vi "Demo - QuickDrop.vi"() -> ()   [LabVIEW 2020]
uses:
  <vilib>/ErrorRing/Error Ring.xnode
  <vilib>/Analysis/NI_AALBase.lvlib
panel:
  in  "error in (no error) 2":errorcluster
  out "error out 7":errorcluster
  in  "Numeric 4":dbl
  in  "String 4":string
  out "Numeric 3":dbl
  out "String 3":string
  out "error out 6":errorcluster
  out "error out 5":errorcluster
  out "error out 4":errorcluster
  out "error out 3":errorcluster
  out "error out 2":errorcluster
  out "String 2":string
  out "Numeric 2":dbl
  in  "String":string
  in  "Numeric":dbl
  out "error out":errorcluster
  in  "error in (no error)":errorcluster
  # "LabVIEW QuickDrop"
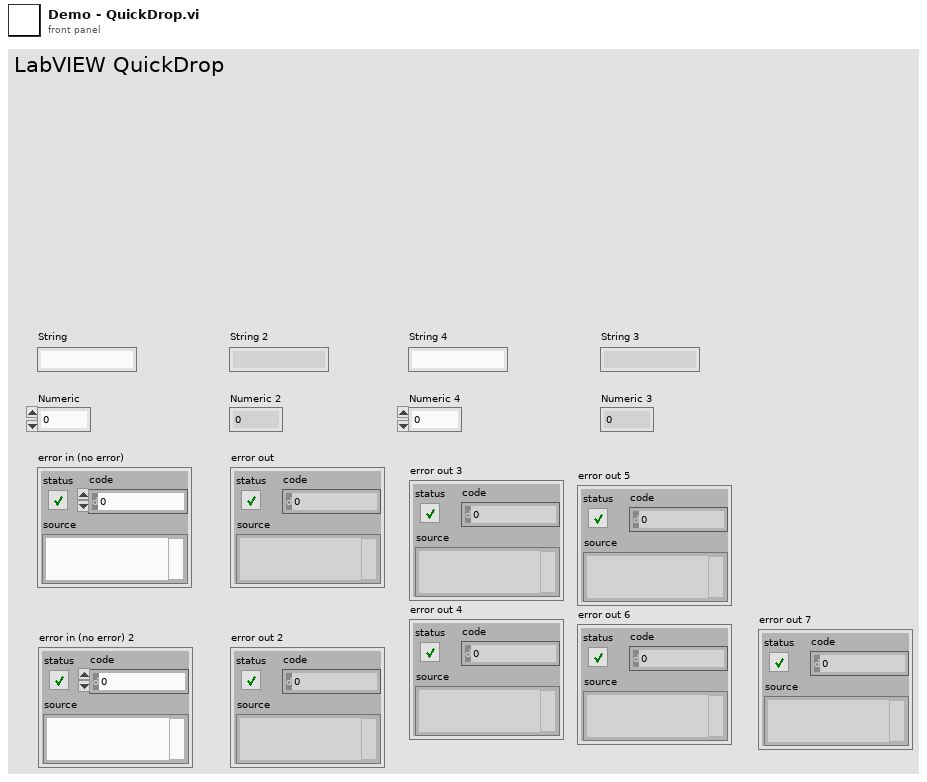
[diagram p1: front panel]
types:
  T1 = enum16{"QD - Wire ctrl & ind", "QD - Wire constants", "QD - FP Reorder as pane connector", "QD - Wire multiple lines", "QD - Wire multiple and cleanup", "QD - Remove item", "QD - Remove unconnected items from bbn", "QD - Reposition labels and icons", "QD - Replace items", "QD - Insert one wire or all wires", "QD - VI Server class rename", "QD - Property method selection", "QD - FP BD to Origin", "QD - Icon Creation", "QD- Combination - Replacing td controls FP", "QD- Combination - Replacing td controls BD"}
  T2 = cluster{"Num 1":i32, "Num 2":i32, "Num 3":i32, "Num 4":i32, "Num 5":i32}
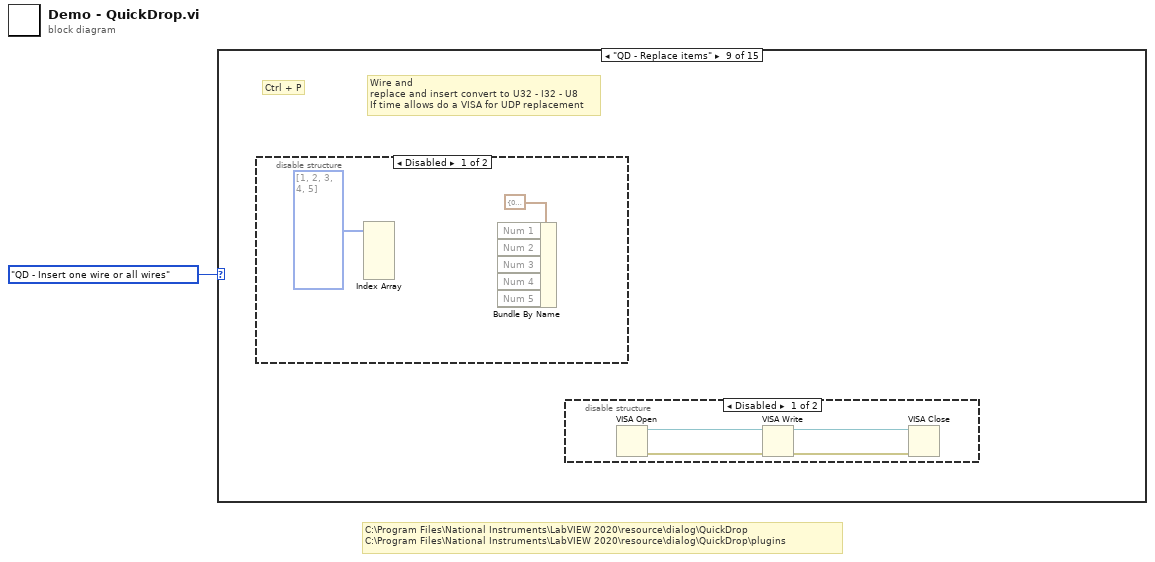
[diagram p0: block diagram]
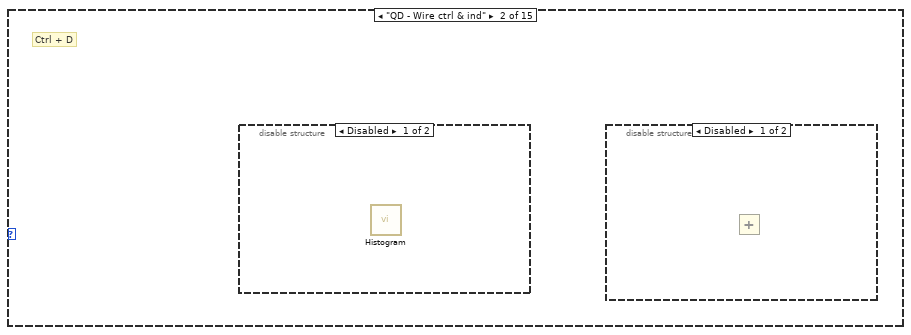
[diagram p3: hidden frame]
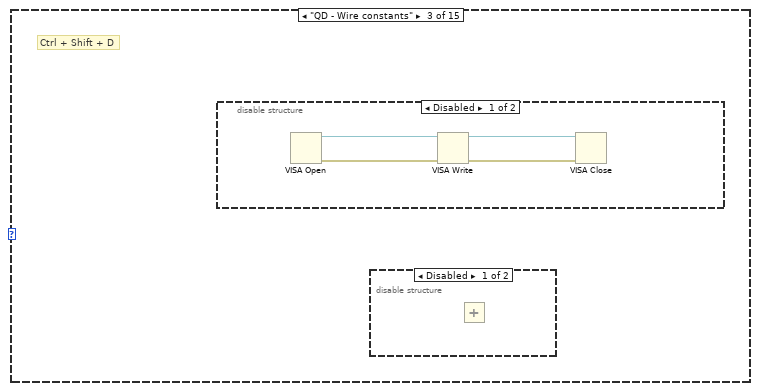
[diagram p6: hidden frame]
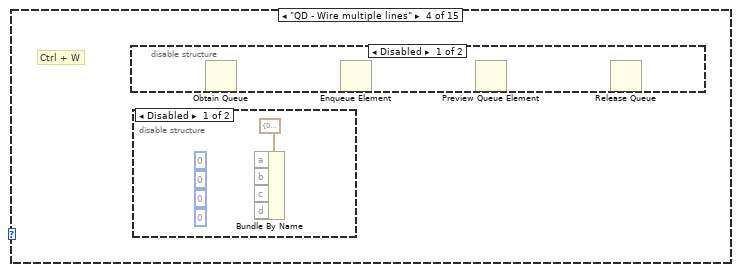
[diagram p9: hidden frame]
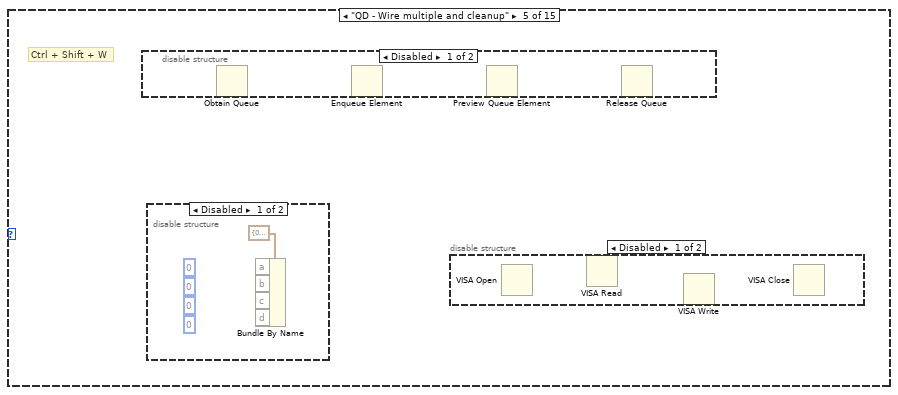
[diagram p12: hidden frame]
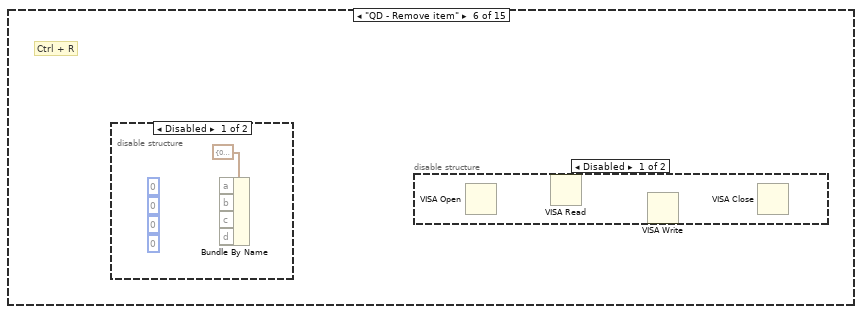
[diagram p16: hidden frame]
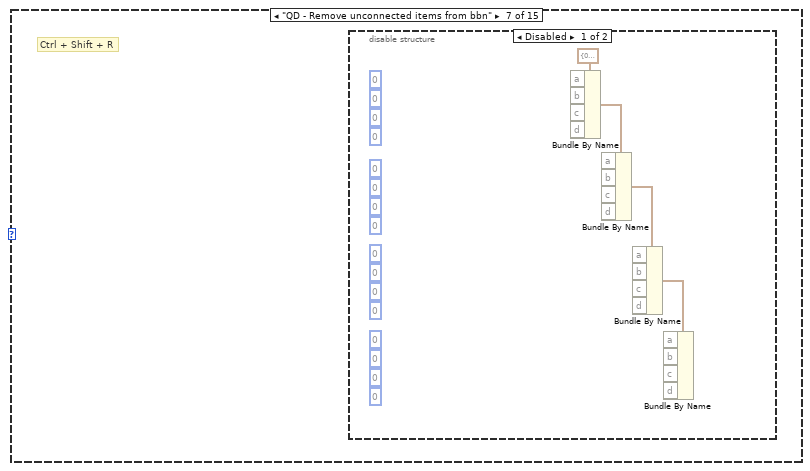
[diagram p19: hidden frame]
diagram:
  # "C:\\Program Files\\National Instruments\\LabVIEW 2020\\resource\\dialog\\QuickDrop\nC:\\Program Files\\National Instruments\\LabVIEW 2020\\resource\\dialog\\QuickDrop\\plugins"
  n1 = case shown="\"QD - Replace items\"" T1."QD - Insert one wire or all wires" {
    frame Default {
      # "Nothing to DEMO"
    }
    frame "QD - Wire ctrl & ind" {
      # "Ctrl + D"
      n2 = disable-structure shown="Disabled" {
        frame Disabled {
          n3 = call <vilib>:"Histogram.vi"() -> ()  [unwired: 8 in, 4 out]
        }
        frame Enabled {
        }
      }
      n4 = disable-structure shown="Disabled" {
        frame Disabled {
          n5 = Add() -> ()  [unwired: 2 in, 1 out]
        }
        frame Enabled {
        }
      }
    }
    frame "QD - Wire constants" {
      # "Ctrl + Shift + D"
      n6 = disable-structure shown="Disabled" {
        frame Disabled {
          n7 = VISA Open() -> (VISA resource name=w5:refnum<visa-resource-name>, error out=w4:errorcluster)  [unwired: 5 in]
          n8 = VISA Write(VISA resource name=w5, error in (no error)=w4) -> (VISA resource name out=w3:refnum<visa-resource-name>, error out=w2:errorcluster)  [unwired: 1 in, 1 out]
          n9 = VISA Close(VISA resource name=w3, error in (no error)=w2) -> ()  [unwired: 1 out]
        }
        frame Enabled {
        }
      }
      n10 = disable-structure shown="Disabled" {
        frame Disabled {
          n11 = Add() -> ()  [unwired: 2 in, 1 out]
        }
        frame Enabled {
        }
      }
    }
    frame "QD - Wire multiple lines" {
      # "Ctrl + W"
      n12 = disable-structure shown="Disabled" {
        frame Disabled {
          n13 = Obtain Queue() -> ()  [unwired: 5 in, 3 out]
          n14 = Enqueue Element() -> ()  [unwired: 4 in, 3 out]
          n15 = Preview Queue Element() -> ()  [unwired: 3 in, 4 out]
          n16 = Release Queue() -> ()  [unwired: 3 in, 3 out]
        }
        frame Enabled {
        }
      }
      n17 = disable-structure shown="Disabled" {
        frame Disabled {
          (unwired) 0
          (unwired) 0
          (unwired) 0
          (unwired) 0
          n18 = Bundle By Name(cluster=cluster{"a":i32, "b":i32, "c":i32, "d":i32} {"a"=0, "b"=0, "c"=0, "d"=0}) -> ()  [unwired: 4 in, 1 out]
        }
        frame Enabled {
        }
      }
    }
    frame "QD - Wire multiple and cleanup" {
      # "Ctrl + Shift + W"
      n19 = disable-structure shown="Disabled" {
        frame Disabled {
          n20 = Obtain Queue() -> ()  [unwired: 5 in, 3 out]
          n21 = Enqueue Element() -> ()  [unwired: 4 in, 3 out]
          n22 = Preview Queue Element() -> ()  [unwired: 3 in, 4 out]
          n23 = Release Queue() -> ()  [unwired: 3 in, 3 out]
        }
        frame Enabled {
        }
      }
      n24 = disable-structure shown="Disabled" {
        frame Disabled {
          (unwired) 0
          (unwired) 0
          (unwired) 0
          (unwired) 0
          n25 = Bundle By Name(cluster=cluster{"a":i32, "b":i32, "c":i32, "d":i32} {"a"=0, "b"=0, "c"=0, "d"=0}) -> ()  [unwired: 4 in, 1 out]
        }
        frame Enabled {
        }
      }
      n26 = disable-structure shown="Disabled" {
        frame Disabled {
          n27 = VISA Open() -> ()  [unwired: 5 in, 2 out]
          n28 = VISA Read() -> ()  [unwired: 3 in, 4 out]
          n29 = VISA Write() -> ()  [unwired: 3 in, 3 out]
          n30 = VISA Close() -> ()  [unwired: 2 in, 1 out]
        }
        frame Enabled {
        }
      }
    }
    frame "QD - Remove item" {
      # "Ctrl + R"
      n31 = disable-structure shown="Disabled" {
        frame Disabled {
          (unwired) 0
          (unwired) 0
          (unwired) 0
          (unwired) 0
          n32 = Bundle By Name(cluster=cluster{"a":i32, "b":i32, "c":i32, "d":i32} {"a"=0, "b"=0, "c"=0, "d"=0}) -> ()  [unwired: 4 in, 1 out]
        }
        frame Enabled {
        }
      }
      n33 = disable-structure shown="Disabled" {
        frame Disabled {
          n34 = VISA Open() -> ()  [unwired: 5 in, 2 out]
          n35 = VISA Read() -> ()  [unwired: 3 in, 4 out]
          n36 = VISA Write() -> ()  [unwired: 3 in, 3 out]
          n37 = VISA Close() -> ()  [unwired: 2 in, 1 out]
        }
        frame Enabled {
        }
      }
    }
    frame "QD - Remove unconnected items from bbn" {
      # "Ctrl + Shift + R"
      n38 = disable-structure shown="Disabled" {
        frame Disabled {
          (unwired) 0
          (unwired) 0
          (unwired) 0
          (unwired) 0
          (unwired) 0
          (unwired) 0
          (unwired) 0
          (unwired) 0
          (unwired) 0
          (unwired) 0
          (unwired) 0
          (unwired) 0
          (unwired) 0
          (unwired) 0
          (unwired) 0
          (unwired) 0
          n39 = Bundle By Name(cluster=cluster{"a":i32, "b":i32, "c":i32, "d":i32} {"a"=0, "b"=0, "c"=0, "d"=0}) -> (w9:cluster{"a":i32, "b":i32, "c":i32, "d":i32})  [unwired: 4 in]
          n40 = Bundle By Name(cluster=w9) -> (w10:cluster{"a":i32, "b":i32, "c":i32, "d":i32})  [unwired: 4 in]
          n41 = Bundle By Name(cluster=w10) -> (w11:cluster{"a":i32, "b":i32, "c":i32, "d":i32})  [unwired: 4 in]
          n42 = Bundle By Name(cluster=w11) -> ()  [unwired: 4 in, 1 out]
        }
        frame Enabled {
        }
      }
    }
    frame "QD - Reposition labels and icons" {
      # "Ctrl + T"
      n43 = disable-structure shown="Disabled" {
        frame Disabled {
        }
        frame Enabled {
        }
      }
      n44 = disable-structure shown="Disabled" {
        frame Disabled {
          # "Do it with different config position"
        }
        frame Enabled {
        }
      }
    }
    frame "QD - Replace items" {
      # "Ctrl + P"
      # "Wire and \nreplace and insert convert to U32 - I32 - U8\nIf time allows do a VISA for UDP replacement"
      n45 = disable-structure shown="Disabled" {
        frame Disabled {
          n46 = Index Array(array=u32[] [1, 2, 3, 4, 5]) -> ()  [unwired: 5 in, 5 out]
          n47 = Bundle By Name(cluster=T2 {"Num 1"=0, "Num 2"=0, "Num 3"=0, "Num 4"=0, "Num 5"=0}) -> ()  [unwired: 5 in, 1 out]
        }
        frame Enabled {
        }
      }
      n48 = disable-structure shown="Disabled" {
        frame Disabled {
          n49 = VISA Open() -> (VISA resource name=w16:refnum<visa-resource-name>, error out=w15:errorcluster)  [unwired: 5 in]
          n50 = VISA Write(VISA resource name=w16, error in (no error)=w15) -> (VISA resource name out=w14:refnum<visa-resource-name>, error out=w13:errorcluster)  [unwired: 1 in, 1 out]
          n51 = VISA Close(VISA resource name=w14, error in (no error)=w13) -> ()  [unwired: 1 out]
        }
        frame Enabled {
        }
      }
    }
    frame "QD - VI Server class rename" {
      # "Ctrl + B"
      # "VI Server Class ------ B\nApplication\nProject\nPane\nVI\nArray\nCluster\nListbox"
      n52 = disable-structure shown="Disabled" {
        frame Disabled {
          n53 = property class="App" props=["Name"]() -> ()  [unwired: 2 in, 3 out]
        }
        frame Enabled {
        }
      }
    }
    frame "QD - Property method selection" {
      # "Ctrl + Shift + B"
      # "Properties and methods ------ Shift + B -\nFront Panel\nPath\nLibrary\nVI Name"
      n54 = disable-structure shown="Disabled" {
        frame Disabled {
          n55 = property class="VI" props=[]() -> ()  [unwired: 2 in, 3 out]
        }
        frame Enabled {
        }
      }
    }
    frame "QD - FP Reorder as pane connector" {
      # "Ctrl + F"
      # "Do it in a new VI"
    }
    frame "QD - FP BD to Origin" {
      # "Ctrl + O"
    }
    frame "QD - Icon Creation" {
      # "Ctrl + K"
    }
    frame "QD - Insert one wire or all wires" {
      # "Ctrl + I"
      # "Ctrl + Shift + I"
      # "Constructor Node\n  System 4.0.0.0\n  System.Net.NetworkInformation\n  Ping\ncr\nwire \nAdd Constructor \n    System.Net\n   IP Address\nThen insert .net rn and nv"
      # "Insert stall VI to all of them"
      # "crf\ncf\n\nInsert \nrtf\nrn"
      n56 = xnode "Error Ring"() -> ("error out"=→"error out 2":errorcluster)
      n57 = xnode "Error Ring"() -> ("error out"=→"error out 3":errorcluster)
      n58 = xnode "Error Ring"() -> ("error out"=→"error out 4":errorcluster)
      n59 = xnode "Error Ring"() -> ("error out"=→"error out 5":errorcluster)
      n60 = xnode "Error Ring"() -> ("error out"=→"error out 6":errorcluster)
    }
  }
